vi "Run.vi"(8 "error in (no error)":errorcluster, 11 "CorrFactor in":refnum<class "CorrFactor.lvclass">) -> (0 "error out":errorcluster, 2 "TimeOut":bool, 3 "CorrFactor out":refnum<class "CorrFactor.lvclass">)   [LabVIEW 2018, in "AnalysisPlugins.lvlib" / "CorrFactor.lvclass"]
uses:
  CorrFactor.lvclass
  F:/Projects/ICDAS/NistPluggableModules/Analysis/AnalysisPlugins/AnalysisPluginBaseClass/AnalysisPluginsBase.lvclass
  Typedefs/clAnalysisConfig.ctl
  Typedefs/3458 Params.ctl
  AnalysisPluginBaseClass/AnalysisPluginsBase.lvclass/AnalysisPluginsBase.ctl
  AnalysisPluginBaseClass/Accessors/Read AnalysisConfig.vi
panel:
  out "Averages":T1={"Vin(s) (Vrms)"=[66.5464683124677], "Vin phase(s) (deg)"=[0.0], "Vin Freq. (Hz)"=65.0} {"Vin(s) (Vrms)" format="%.7e"; "Vin phase(s) (deg)" format="%.7e"; "Vin Freq. (Hz)" format="%.7f"}
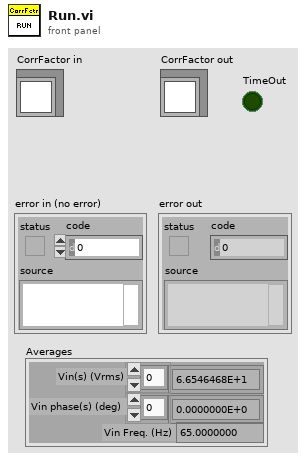
[diagram p1: front panel]
types:
  T1 = cluster{"Vin(s) (Vrms)":dbl[], "Vin phase(s) (deg)":dbl[], "Vin Freq. (Hz)":dbl}
  T2 = typedef "AnalysisPlugins.lvlib/CorrFactor.lvclass/clAnalysisConfig.ctl" = cluster{"HP 3458 address":string, "Amplitude":dbl, "3458  Params:":T3}
  T3 = typedef "AnalysisPlugins.lvlib/CorrFactor.lvclass/3458 Params.ctl" = cluster{"Record Size":i32, "Input Freq (Hz)":dbl, "# Cycles (Desired)":dbl, "Sampling Mode:":u16, "# of Record Avgs./Meas.":i32, "Trigger Mode":u16, "Trig. Level (%)":dbl, "# of Meas. Runs":i32, "Trigger Slope":u16}
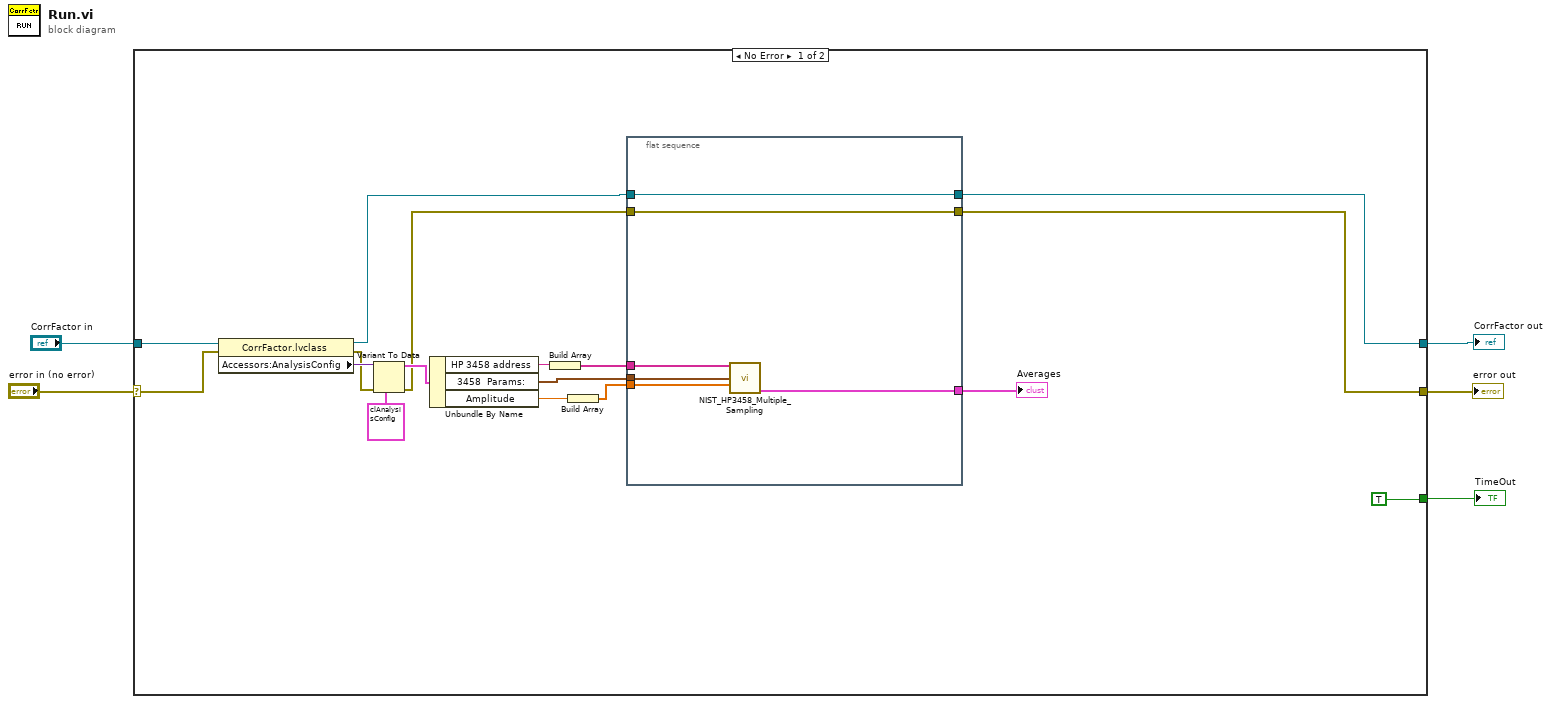
[diagram p0: block diagram]
diagram:
  n1 = case shown="No Error" "error in (no error)" {
    selector: "error in (no error)" -> [w21 w29]
    tunnel: "CorrFactor in" -> [w22 w30]
    tunnel: [w8 w30] -> w3
    tunnel: [w6 w29] -> w2
    tunnel: [TRUE _] -> w1
    frame No Error {
      n2 = property class="CorrFactor.lvclass"(reference=w22, error in=w21) -> (reference out=w9:refnum<class "CorrFactor.lvclass">, error out=w18:errorcluster, "Accessors:AnalysisConfig"=w20:variant)
      n3 = Variant To Data(error in=w18, type=T2 {"HP 3458 address"="", "Amplitude"=0.0, "3458  Params:"={"Record Size"=4096, "Input Freq (Hz)"=50.0, "# Cycles (Desired)"=501.0, "Sampling Mode:"=1, "# of Record Avgs./Meas."=1, "Trigger Mode"=0, "Trig. Level (%)"=0.0, "# of Meas. Runs"=5, "Trigger Slope"=0}} ("clAnalysisConfig"), Variant=w20) -> (data=w17:T2, error out=w7:errorcluster)
      n4 = Unbundle By Name(w17) -> ("HP 3458 address"=w16:string, "3458  Params:"=w14:T3, "Amplitude"=w13:dbl)
      n5 = Build Array(w16) -> (w15:string[])
      n6 = Build Array(w13) -> (w12:dbl[])
      n7 = flat-sequence {
        tunnel: w15 -> [w28]
        tunnel: w14 -> [w27]
        tunnel: w12 -> [w26]
        tunnel: [w25] -> w11
        tunnel: w9 -> [w24]
        tunnel: [w24] -> w8
        tunnel: w7 -> [w23]
        tunnel: [w23] -> w6
        frame #0 {
          n8 = call "NIST_HP3458_Multiple_Sampling.vi"("HP3458 Address(s):"=w28, "Input Sampling Parameters:"=w27, "HP3458 Input Voltage(s) (Vrms):"=w26) -> ("Averages"=w25:T1)  [unwired: 9 in, 3 out]
        }
      }
      "Averages" <- w11
    }
    frame Error {
    }
  }
  "error out" <- w2
  "CorrFactor out" <- w3
  "TimeOut" <- w1
